vi "Low_Power_CH2.vi"(8 "Modulation parameter":T1, 9 "output bits":i8[](array[numeric]), 10 "Boolean":bool, 11 "Record BER":bool) -> (3 "subarray2":i8[](array[numeric]))   [LabVIEW 2022 SP3]
panel:
  out "No. Bits LP":dbl
  out "?":T1
  out "Low-Power Decoded Message":string
  in  "Expected message LP":string="Non Critical Data\nNon Critical Data\nNon Critical Data\nNon Critical Data\nNon Critical Data"
  out "Acum. Err LP":dbl
  out "Acc. BER LP":dbl format="%#_4g"
  out "Inst. BER LP":dbl format="%#_4g"
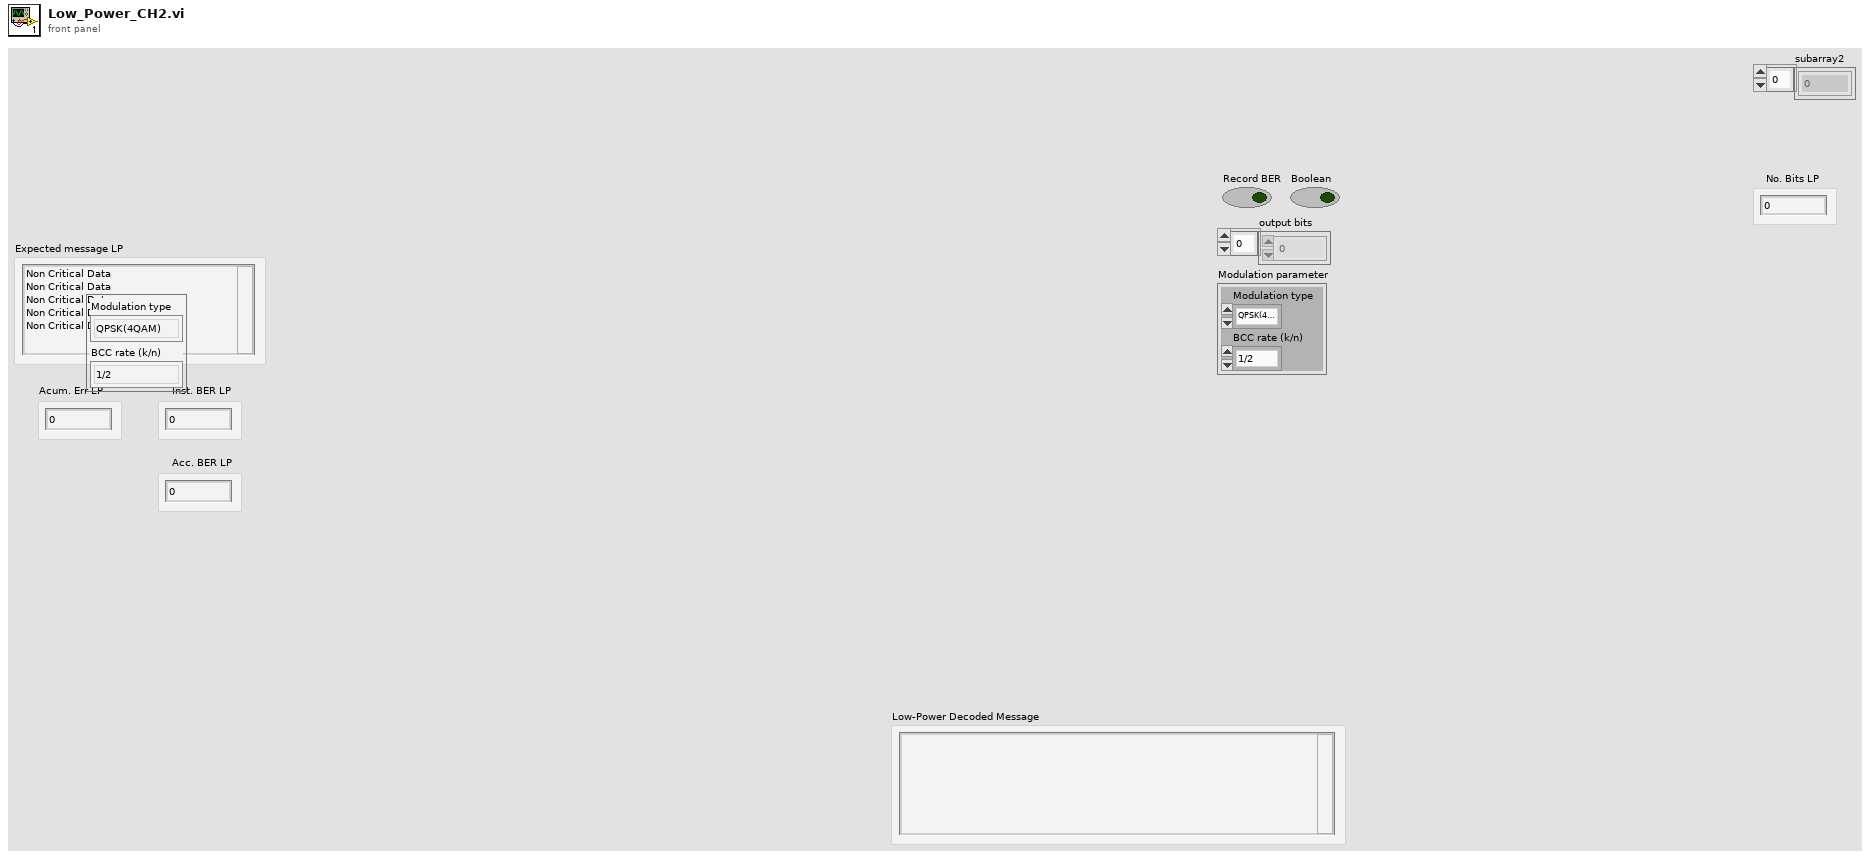
[diagram p1: front panel]
types:
  T1 = cluster{"Modulation type":enum16{"QPSK(4QAM)", "64QAM", "16QAM", "BPSK"}, "BCC rate (k/n)":enum16{"1/2", "2/3", "3/4"}}
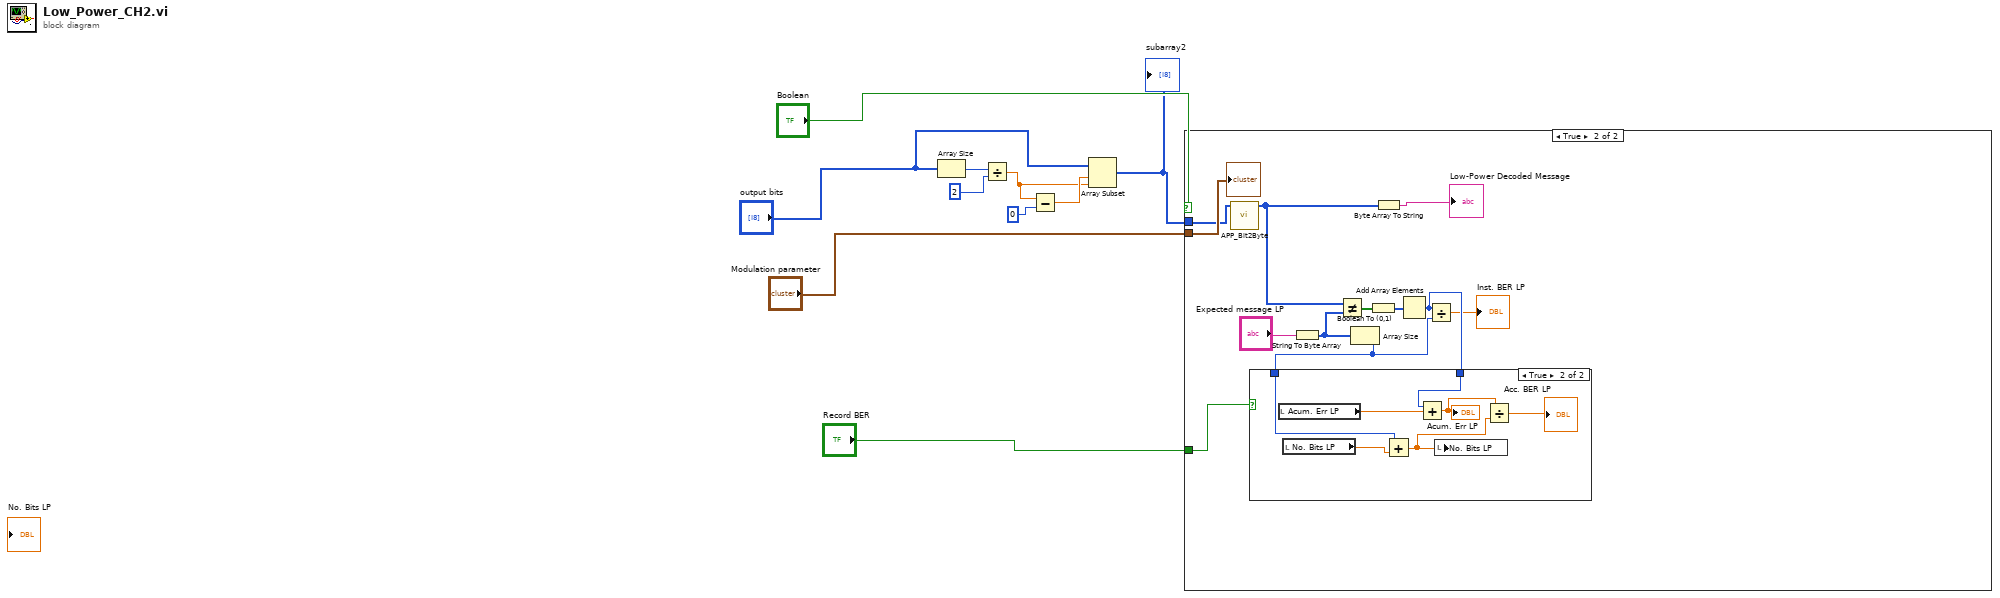
[diagram p0: block diagram]
diagram:
  n1 = Array Size(array="output bits") -> (size(s)=w7:i32)
  n2 = Divide(x=w7, y=2) -> (x/y=w2:dbl)
  n3 = Subtract(x=w2, y=0) -> (x-y=w3:dbl)
  n4 = Array Subset(array="output bits", index=w3, length=w2) -> (w1:i8[])
  "subarray2" <- w1
  n5 = case shown="True" "Boolean" {
    tunnel: "Modulation parameter" -> [_ w22]
    tunnel: "Record BER" -> [_ w13]
    tunnel: w1 -> [_ w11]
    frame False {
    }
    frame True {
      n6 = call "APP_Bit2Byte.vi"("input bit stream"=w11) -> ("output byte stream"=w15:u8[])  [unwired: 10 in]
      n7 = String To Byte Array(string="Expected message LP") -> (unsigned byte array=w19:u8[])
      n8 = Not Equal?(x=w15, y=w19) -> (x != y?=w17:bool[])
      n9 = Array Size(array=w19) -> (size(s)=w20:i32)
      n10 = Boolean To (0,1)(Boolean=w17) -> (0, 1=w16:i16[])
      n11 = Byte Array To String(unsigned byte array=w15) -> (string=→"Low-Power Decoded Message":string)
      n12 = Add Array Elements(numeric array=w16) -> (sum=w14:i16)
      n13 = case shown="True" w13 {
        tunnel: w20 -> [_ w28]
        tunnel: w14 -> [_ w26]
        frame False {
        }
        frame True {
          n14 = local read "Acum. Err LP"() -> (w27:dbl)
          n15 = local read "No. Bits LP"() -> (w29:dbl)
          n16 = Add(x=w28, y=w29) -> (x+y=w23:dbl)
          n17 = Add(x=w26, y=w27) -> (x+y=w25:dbl)
          "Acum. Err LP" <- w25
          n18 = local write "No. Bits LP"(w23) -> ()
          n19 = Divide(x=w25, y=w23) -> (x/y=→"Acc. BER LP":dbl)
        }
      }
      n20 = Divide(x=w14, y=w20) -> (x/y=→"Inst. BER LP":dbl)
      "?" <- w22
    }
  }
